vi "Projecte 1.1.vi"() -> ()   [LabVIEW 2014]
uses:
  <vilib>/LabVIEW Hacker/LINX/Public/Peripherals/PWM/Set Duty Cycle 1 Chan.vi
  <vilib>/LabVIEW Hacker/LINX/Public/Peripherals/Analog/Analog Read 1 Chan.vi
  <vilib>/LabVIEW Hacker/LINX/LVH-LINX.lvlib
panel:
  in  "access (0:read/write)":enum16{"read/write", "read-only", "write-only"}(ring)
  in  "operation (0:open)":T1(ring)
  in  "file path (use dialog)":path
  out "Error Out":errorcluster
  in  "Serial Port":refnum<visa-resource-name>="N/A"
  out "V1 temps real":cluster{"Y":dbl[], "Y":dbl[]}[](graph)
  out "duty cycle":dbl
  in  "Mesures":i32
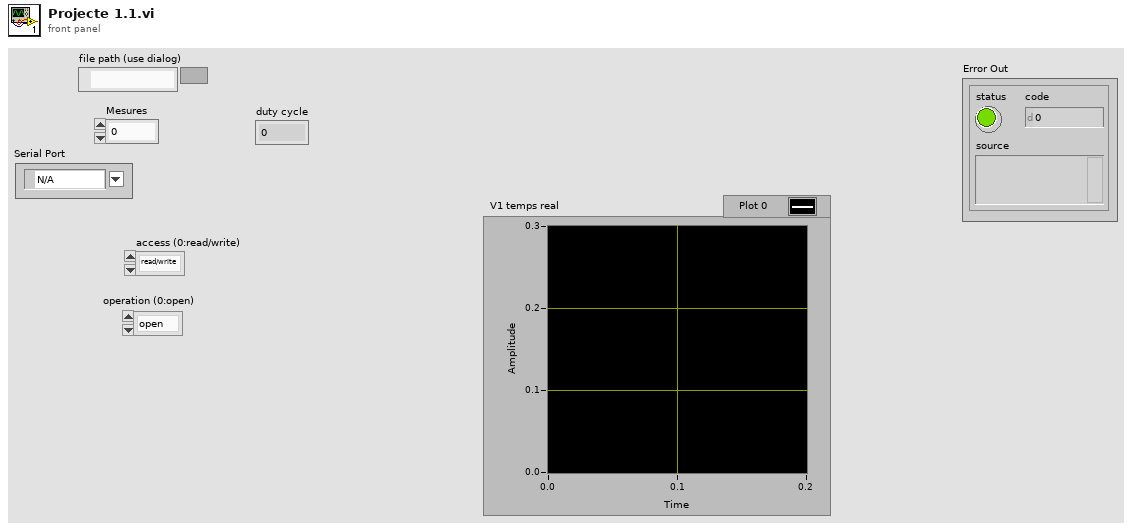
[diagram p1: front panel]
types:
  T1 = enum16{"open", "replace", "create", "open or create", "replace or create", "replace or create with confirmation"}
  T2 = typedef "LVH-LINX.lvlib/LINX Ref.ctl" = cluster{"Platform":T3, "Interface":T4, "LINX Device Config":T5}
  T3 = typedef "LVH-LINX.lvlib/Platform.ctl" = enum16{"LINX", "myRIO"}
  T4 = typedef "LVH-LINX.lvlib/Interface.ctl" = enum16{"Serial", "TCP"}
  T5 = typedef "LVH-LINX.lvlib/Device.lvlib/LINX Device Config.ctl" = cluster{"Interface":T4, "COM Port":refnum<visa-resource-name>, "TCP Configuration":T6, "Device Family":T7, "Device ID":u8, "Device Name":string, "TCP Ref":refnum<k5>}
  T6 = typedef "LVH-LINX.lvlib/Device.lvlib/TCP Config.ctl" = cluster{"IP Address":string, "Port":u16}
  T7 = typedef "LVH-LINX.lvlib/Device Family.ctl" = enum8{"National Instruments", "Digilent", "Arduino"}
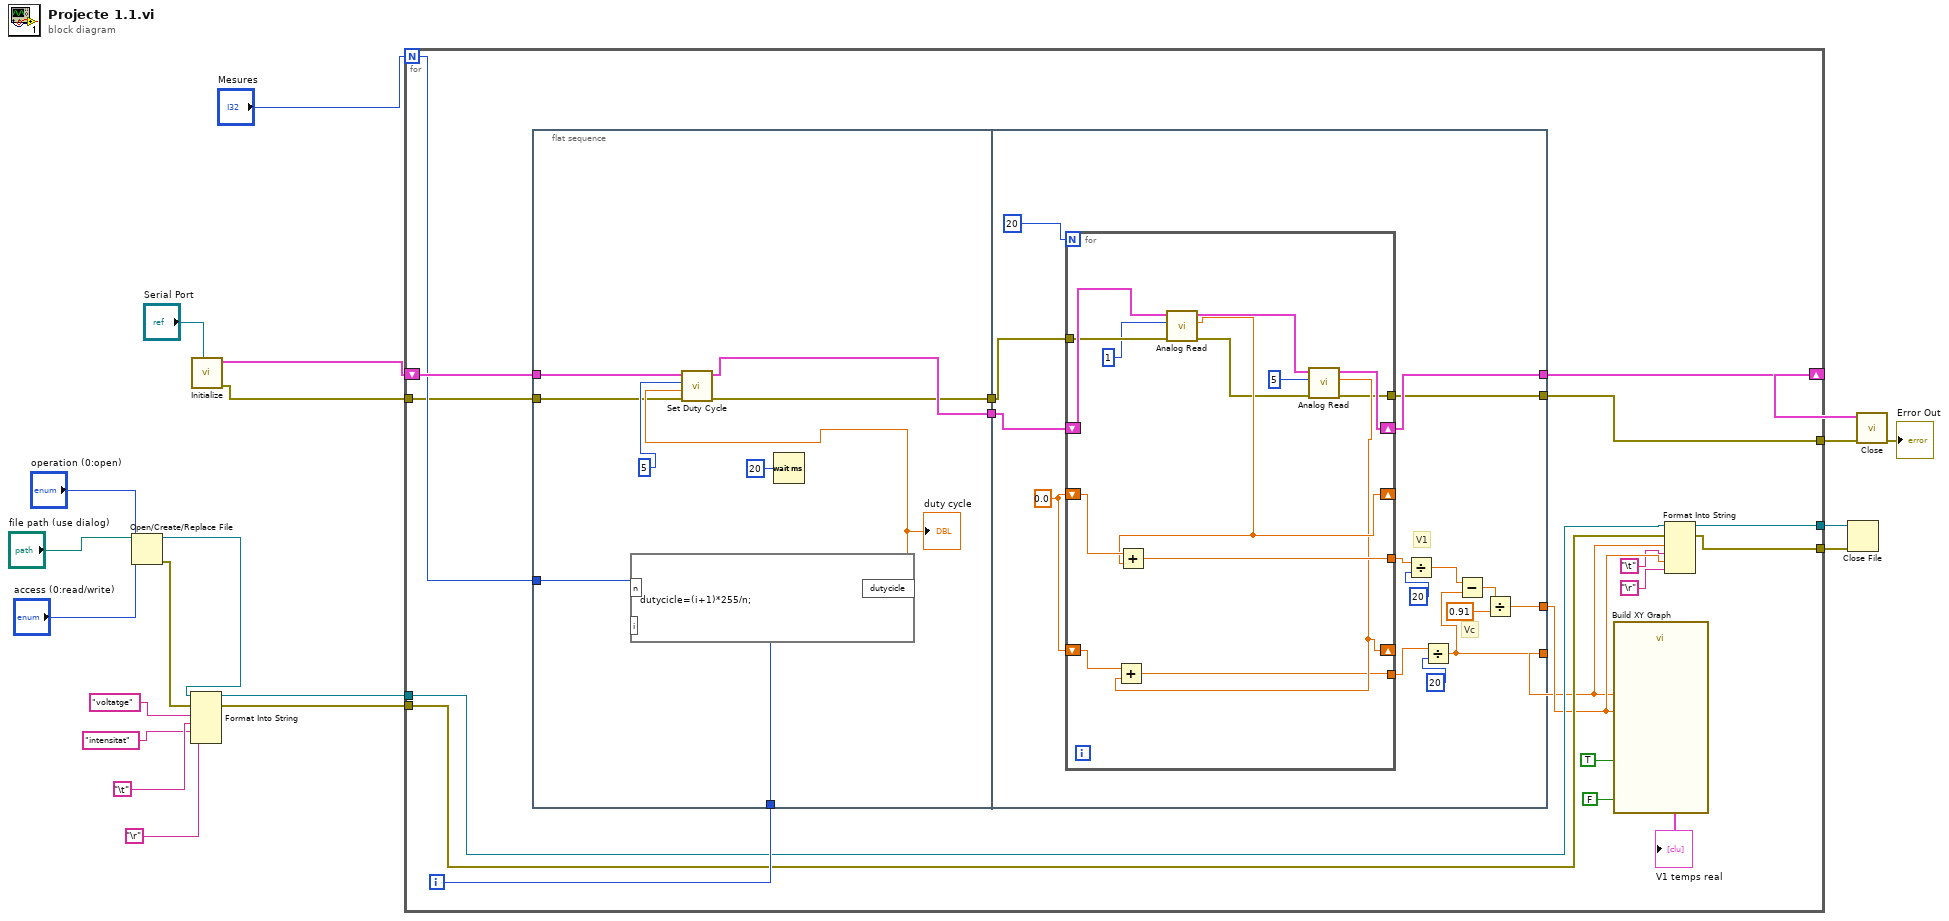
[diagram p0: block diagram]
diagram:
  n1 = Open/Create/Replace File(file path (use dialog)="file path (use dialog)", operation (0:open)="operation (0:open)", access (0:read/write)="access (0:read/write)") -> (refnum out=w6:refnum<file>, error out=w4:errorcluster)  [unwired: 3 in, 1 out]
  n2 = Format Into String(initial string=w6, error in=w4, "voltatge" ("String"), "\t", "intensitat" ("String"), "\r") -> (resulting string=w5:refnum<file>, error out=w3:errorcluster)  [unwired: 1 in]
  n3 = call <vilib>:"Initialize.vi"("Serial Port"="Serial Port") -> ("Error Out"=w16:errorcluster, "LINX Ref"=w20:T2)  [unwired: 8 in, 1 out]
  n4 = for {
    N: "Mesures" -> [w36]
    shift-right: [w35] -> w18
    shift-left: w20 -> [w38]
    tunnel: w16 -> [w33]
    tunnel: [w31] -> w15
    tunnel: w5 -> [w28]
    tunnel: w3 -> [w27]
    tunnel: [w26] -> w2
    tunnel: [w25] -> w1
    i -> [w34]
    n5 = flat-sequence {
      tunnel: w38 -> [w46]
      tunnel: [w47] -> w37
      tunnel: w36 -> [w43]
      tunnel: w34 -> [w42]
      tunnel: w33 -> [w41]
      tunnel: [w40] -> w32
      tunnel: w37 -> [w57]
      tunnel: [w56] -> w35
      tunnel: [w50] -> w23
      tunnel: [w53] -> w24
      tunnel: w32 -> [w52]
      tunnel: [w51] -> w31
      frame #0 {
        n6 = formula code="dutycicle=(i+1)*255/n;"("i"=w42, "n"=w43) -> ("dutycicle"=w45:dbl)
        "duty cycle" <- w45
        n7 = call-poly <vilib>:"Set Duty Cycle.vi"("Error In"=w41, "Duty Cycle"=w45, "PWM Channel"=u8 5, "LINX Resource"=w46) -> ("Error Out"=w40:errorcluster, "LINX Resource"=w47:T2)  [unwired: 6 in]
        n8 = Wait (ms)(milliseconds to wait=u32 20) -> ()  [unwired: 1 out]
      }
      frame #1 {
        w60 = 0.0
        # "Vc"
        # "V1"
        n9 = for {
          N: 20 -> [_]
          shift-right: [w68] -> w56
          shift-left: w57 -> [w77]
          shift-right: [w72] -> _
          shift-left: w60 -> [w74]
          tunnel: [w73] -> w62
          shift-right: [w70] -> _
          shift-left: w60 -> [w71]
          tunnel: [w69] -> w58
          tunnel: w52 -> [w67]
          tunnel: [w65] -> w51
          n10 = call-poly <vilib>:"Analog Read.vi"("Error In"=w67, "Analog Channel"=u8 1, "LINX Resource"=w77) -> ("Error Out"=w66:errorcluster, "AI Value"=w72:dbl, "LINX Resource"=w75:T2)  [unwired: 5 in, 1 out]
          n11 = Add(x=w74, y=w72) -> (x+y=w73:dbl)
          n12 = call-poly <vilib>:"Analog Read.vi"("Error In"=w66, "Analog Channel"=u8 5, "LINX Resource"=w75) -> ("Error Out"=w65:errorcluster, "AI Value"=w70:dbl, "LINX Resource"=w68:T2)  [unwired: 5 in, 1 out]
          n13 = Add(x=w71, y=w70) -> (x+y=w69:dbl)
        }
        n14 = Divide(x=w62, y=20) -> (x/y=w49:dbl)
        n15 = Divide(x=w58, y=20) -> (x/y=w50:dbl)
        n16 = Subtract(x=w49, y=w50) -> (x-y=w55:dbl)
        n17 = Divide(x=w55, y=0.91) -> (x/y=w53:dbl)
      }
    }
    n18 = call "Build XY Graph"("Enable"=TRUE, "Reset"=FALSE, "Y Input"=w24, "X Input"=w23) -> ("XY Graph"=→"V1 temps real":cluster{"X":dbl[], "Y":dbl[]}[])  [unwired: 6 in, 1 out]
    n19 = Format Into String(initial string=w28, error in=w27, w23, "\t", w24, "\r") -> (resulting string=w26:refnum<file>, error out=w25:errorcluster)  [unwired: 1 in]
  }
  n20 = Close File(refnum=w2, error in=w1) -> ()  [unwired: 2 out]
  n21 = call <vilib>:"Close.vi"("Error In"=w15, "LINX Resource"=w18) -> ("Error Out"=→"Error Out":errorcluster)  [unwired: 8 in, 1 out]
